vi "PID final controller.vi"(4 "e_sum":dbl, 5 "Kp":dbl, 6 "e_t":dbl, 7 "Ki":dbl, 8 "Ts":dbl, 9 "q":dbl, 10 "SP":dbl, 11 "Kd":dbl) -> (1 "sum_out":dbl, 2 "u_out":dbl, 3 "e_out":dbl)   [LabVIEW 2014]
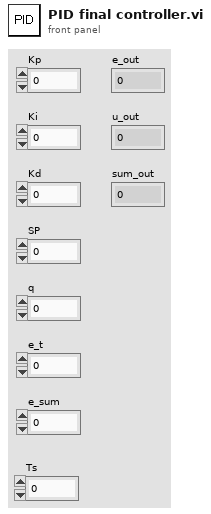
[diagram p1: front panel]
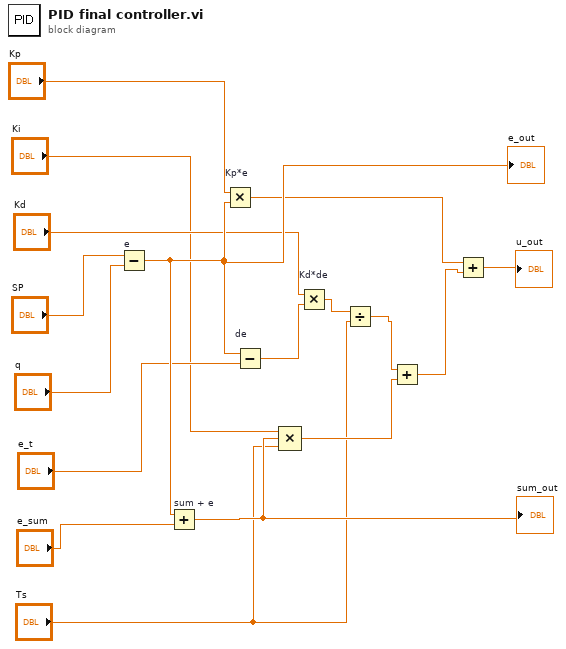
[diagram p0: block diagram]
diagram:
  n1 = Subtract "e"(x="SP", y="q") -> (x-y=w17:dbl)
  "e_out" <- w17
  n2 = Add "sum + e"(x=w17, y="e_sum") -> (x+y=w5:dbl)
  "sum_out" <- w5
  n3 = Multiply "Kp*e"(x="Kp", y=w17) -> (x*y=w14:dbl)
  n4 = Subtract "de"(x=w17, y="e_t") -> (x-y=w13:dbl)
  n5 = Compound Arithmetic op=MULTIPLY("Ki", w5, "Ts") -> (w4:dbl)
  n6 = Multiply "Kd*de"(x="Kd", y=w13) -> (x*y=w2:dbl)
  n7 = Divide(x=w2, y="Ts") -> (x/y=w3:dbl)
  n8 = Add(x=w3, y=w4) -> (x+y=w15:dbl)
  n9 = Add(x=w14, y=w15) -> (x+y=→"u_out":dbl)
